vi "U6 Stream AIN with Timers & Counters.vi"() -> ()   [LabVIEW 2021]
panel:
  out "UD Backlog [%]":dbl format="%.2f"
  in  "Reset Timer1/Counter1":bool
  out "Combined Counter Data":u32[](array[numeric])
  out "U6 Backlog [%]":dbl format="%.2f"
  out "# Scans Read":i32
  out "# of iterations":i32
  out "Data":dbl[][](array[numeric]) format="%.3f"
  in  "Scan Rate (Hz)":dbl=1000.0 format="%.3f"
  in  "FirstFound":bool=TRUE
  in  "stop":bool
  in  "Address":string="1"
  out "Error Message":string
  # "This example streams AIN0, Timer1 (duty cycle input on\nFIO1), Counter1 (FIO2), and the FIO/EIO digital inputs.\n\nTimer0 is configured as 16-bit PWM output (FIO0).  Frequency\nis 40.7 Hz and duty cycle is 25%.\n\nFor testing, short FIO0 to FIO1 and FIO2."
  # "AIN0               TMR1 (LSW)         TMR1 (MSW)    CNT (LSW)        CNT(MSW)        FIO/EIO"
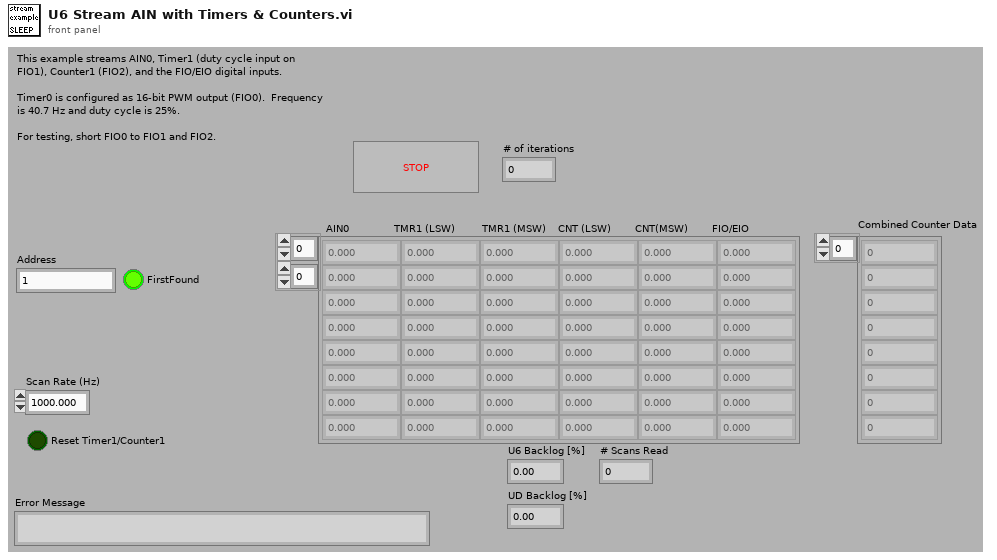
[diagram p1: front panel]
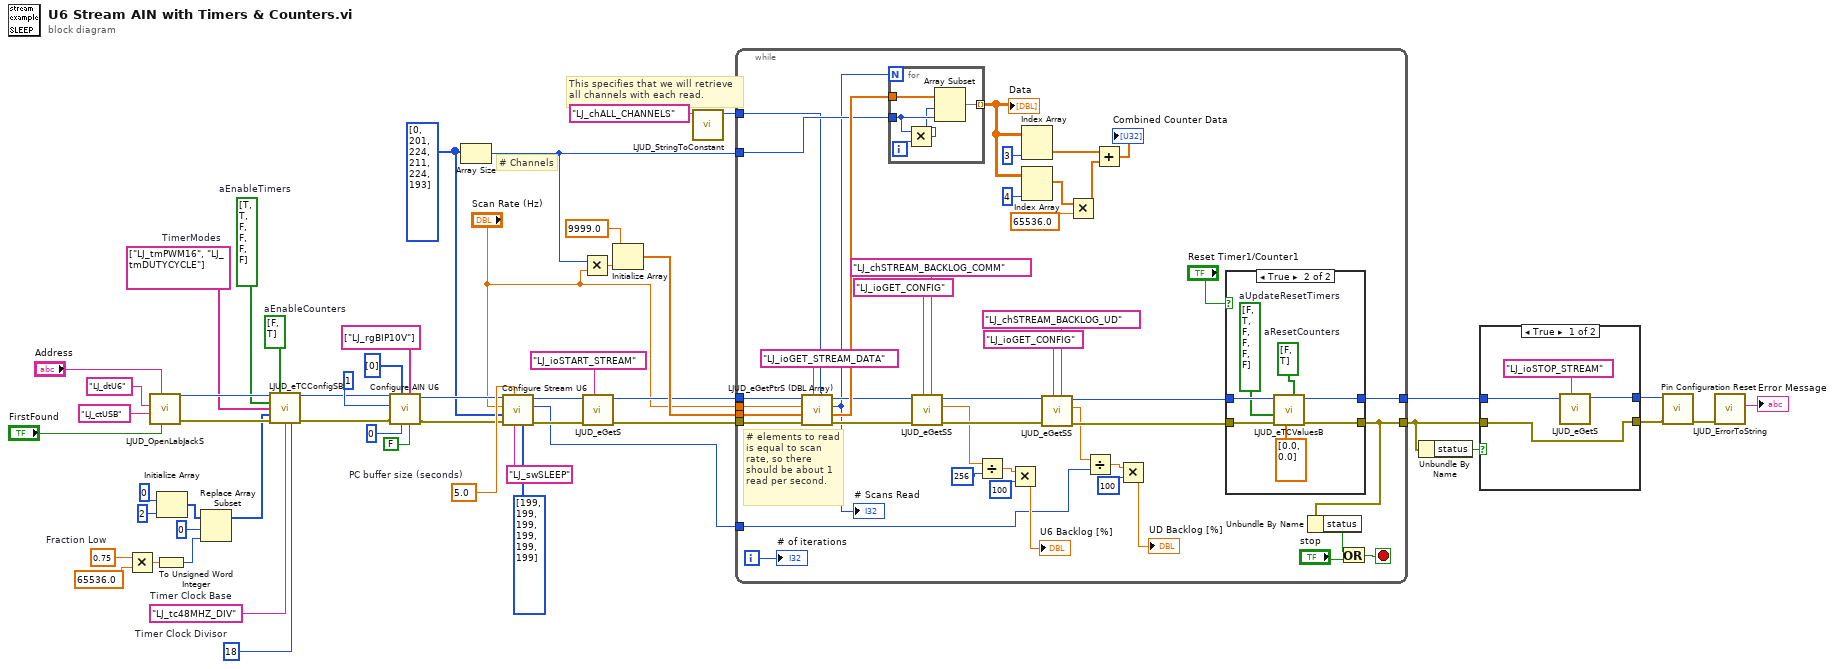
[diagram p0: block diagram]
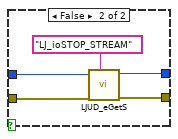
[diagram p3: hidden frame]
diagram:
  w8 = 18  # Timer Clock Divisor
  w9 = "LJ_tc48MHZ_DIV"  # Timer Clock Base
  w12 = bool[] [FALSE, TRUE]  # aEnableCounters
  w14 = 0.75  # Fraction Low
  w10 = string[] ["LJ_tmPWM16", "LJ_tmDUTYCYCLE"]  # TimerModes
  w11 = bool[] [TRUE, TRUE, FALSE, FALSE, FALSE, FALSE]  # aEnableTimers
  w26 = i32[] [0, 201, 224, 211, 224, 193] ("Channels")
  w40 = 5.0  # PC buffer size (seconds)
  # "# Channels"
  # "This specifies that we will retrieve\nall channels with each read."
  n1 = Multiply(x=w14, y=65536.0) -> (x*y=w16:dbl)
  n2 = call "LJUD_OpenLabJackS.vi"("FirstFound"="FirstFound", "Address"="Address", "ConnectionType"="LJ_ctUSB", "DeviceType"="LJ_dtU6") -> ("error out"=w22:errorcluster, "Handle"=w23:i32)  [unwired: 5 in, 1 out]
  n3 = To Unsigned Word Integer(number=w16) -> (unsigned 16bit integer=w15:u16)
  n4 = Initialize Array(u16 0 ("PWM Timer Value"), 2 ("Dimension Size")) -> (w18:u16[])
  n5 = Replace Array Subset(array=w18, new element=w15, index=0 ("Index")) -> (w13:u16[])
  n6 = call "LJUD_eTCConfigSB.vi"("Handle In"=w23, "aEnableCounters"=w12, "aEnableTimers"=w11, "aTimerModes"=w10, "aTimerValues"=w13, "error in"=w22, "TimerClockBase"=w9, "TimerClockDivisor"=w8) -> ("Handle Out"=w25:i32, "error out"=w24:errorcluster)  [unwired: 6 in]
  n7 = call "Configure AIN U6.vi"("Binary"=FALSE, "Ranges"=string[] ["LJ_rgBIP10V"], "SettlingFactor"=0, "Positive Channels"=i32[] [0] ("Channels"), "error in"=w24, "Resolution"=1, "Handle In"=w25) -> ("error out"=w39:errorcluster, "Handle Out"=w38:i32)  [unwired: 3 in]
  n8 = Array Size(array=w26) -> (size(s)=w44:i32)
  n9 = call "Configure Stream U6.vi"("Scan List (-)"=i32[] [199, 199, 199, 199, 199, 199] ("Channels"), "Wait Mode"="LJ_swSLEEP" ("Wait Mode (2)"), "PC buffer size (seconds)"=w40, "error in"=w39, "Scan List (+)"=w26, "Scan Rate (Hz)"="Scan Rate (Hz)", "Handle In"=w38) -> ("error out"=w49:errorcluster, "PC buffer size (samples)"=w1:i32, "Handle Out"=w50:i32)  [unwired: 2 in]
  n10 = Multiply(x=w44, y="Scan Rate (Hz)") -> (x*y=w47:dbl)
  n11 = call "LJUD_eGetS.vi"("IOType"="LJ_ioSTART_STREAM", "error in"=w49, "Handle In"=w50) -> ("error out"=w48:errorcluster, "Handle Out"=w37:i32)  [unwired: 6 in, 1 out]
  n12 = Initialize Array(9999.0, w47) -> (w45:dbl[])
  n13 = call "LJUD_StringToConstant.vi"("String"="LJ_chALL_CHANNELS") -> ("Constant Number"=w32:i32)  [unwired: 9 in, 1 out]
  n14 = while {
    tunnel: w1 -> [w54]
    tunnel: w32 -> [w83]
    tunnel: [w72] -> w35
    tunnel: [w71] -> w42
    tunnel: w44 -> [w89]
    tunnel: w45 -> [w92]
    tunnel: "Scan Rate (Hz)" -> [w90]
    tunnel: w48 -> [w94]
    tunnel: w37 -> [w95]
    i -> [w88]
    stop <- w82 stop-if-true
    # "# elements to read\nis equal to scan\nrate, so there\nshould be about 1\nread per second."
    n15 = call "LJUD_eGetPtrS (DBL Array).vi"("Channel"=w83, "IOType"="LJ_ioGET_STREAM_DATA", "error in"=w94, "DBL Array Write"=w92, "Value"=w90, "Handle In"=w95) -> ("error out"=w86:errorcluster, "DBL Array Read"=w91:dbl[], "Value"=w81:i32, "Handle Out"=w87:i32)  [unwired: 2 in]
    "# Scans Read" <- w81
    n16 = for {
      N: w81 -> [_]
      tunnel: w91 -> [w111]
      tunnel: w89 -> [w110]
      tunnel: [w107] -> w80 mode=indexing
      i -> [w109]
      n17 = Multiply(x=w110, y=w109) -> (x*y=w108:i32)
      n18 = Array Subset(array=w111, index=w108, length=w110) -> (w107:dbl[])
    }
    "Data" <- w80
    n19 = call "LJUD_eGetSS.vi"("Channel"="LJ_chSTREAM_BACKLOG_COMM", "IOType"="LJ_ioGET_CONFIG", "error in"=w86, "Handle In"=w87) -> ("error out"=w66:errorcluster, "Value Read"=w58:dbl, "Handle Out"=w67:i32)  [unwired: 5 in]
    n20 = Divide(x=w58, y=256) -> (x/y=w61:dbl)
    n21 = Multiply(x=w61, y=100) -> (x*y=→"U6 Backlog [%]":dbl)
    n22 = Index Array(array=w80, index (col)=3 ("Disabled Index (col)")) -> (element=w76:dbl[])  [unwired: 1 in]
    n23 = Index Array(array=w80, index (col)=4 ("Disabled Index (col)")) -> (element=w77:dbl[])  [unwired: 1 in]
    n24 = call "LJUD_eGetSS.vi"("Channel"="LJ_chSTREAM_BACKLOG_UD", "IOType"="LJ_ioGET_CONFIG", "error in"=w66, "Handle In"=w67) -> ("error out"=w64:errorcluster, "Value Read"=w55:dbl, "Handle Out"=w65:i32)  [unwired: 5 in]
    n25 = Multiply(x=w77, y=65536.0) -> (x*y=w75:dbl[])
    n26 = Divide(x=w55, y=w54) -> (x/y=w60:dbl)
    n27 = Add(x=w76, y=w75) -> (x+y=→"Combined Counter Data":dbl[])
    n28 = Multiply(x=w60, y=100) -> (x*y=→"UD Backlog [%]":dbl)
    n29 = case shown="True" "Reset Timer1/Counter1" {
      tunnel: w64 -> [w99 w106]
      tunnel: w65 -> [w98 w105]
      tunnel: [w99 w104] -> w72
      tunnel: [w98 w103] -> w71
      frame False {
      }
      frame True {
        w102 = bool[] [FALSE, TRUE]  # aResetCounters
        w101 = bool[] [FALSE, TRUE, FALSE, FALSE, FALSE, FALSE]  # aUpdateResetTimers
        n30 = call "LJUD_eTCValuesB.vi"("aResetCounters"=w102, "aTimerValues Write"=dbl[] [0.0, 0.0], "error in"=w106, "aUpdateResetTimers"=w101, "Handle In"=w105) -> ("error out"=w104:errorcluster, "Handle Out"=w103:i32)  [unwired: 3 in, 2 out]
      }
    }
    n31 = Unbundle By Name(w72) -> ("status"=w96:bool)
    n32 = Or(x=w96, y="stop") -> (x .or. y?=w82:bool)
    "# of iterations" <- w88
  }
  n33 = Unbundle By Name(w35) -> ("status"=w34:bool)
  n34 = case shown="True" w34 {
    tunnel: w42 -> [w114 w119]
    tunnel: [w113 w118] -> w7
    tunnel: w35 -> [w113 w117]
    tunnel: [w112 w116] -> w5
    frame True {
      n35 = call "LJUD_eGetS.vi"("IOType"="LJ_ioSTOP_STREAM", "Handle In"=w114) -> ("Handle Out"=w112:i32)  [unwired: 7 in, 2 out]
    }
    frame False {
      n36 = call "LJUD_eGetS.vi"("IOType"="LJ_ioSTOP_STREAM", "error in"=w117, "Handle In"=w119) -> ("error out"=w118:errorcluster, "Handle Out"=w116:i32)  [unwired: 6 in, 1 out]
    }
  }
  n37 = call "Pin Configuration Reset.vi"("error in"=w7, "Handle In"=w5) -> ("error out"=w6:errorcluster)  [unwired: 8 in, 1 out]
  n38 = call "LJUD_ErrorToString.vi"("error in"=w6) -> ("String"=→"Error Message":string)  [unwired: 10 in]
